vi "ActionVIOnSave.vi"(8 "error in (no error)":errorcluster, 11 "Device Item Ref in":T1 format="%.0x") -> (0 "error out":errorcluster, 3 "Device Item Ref out":T1 format="%.0x")   [LabVIEW 2019, in "Control Addon System Explorer.lvlib"]
uses:
  Control Addon System Explorer.lvlib
  <vilib>/NI VeriStand/Custom Device API/Custom Device Item Ref.ctl
  Types/Action.ctl
  Addon Shared/SubVIs/Constants.vi
  <vilib>/NI VeriStand/Custom Device API/NI VeriStand - Get Item Property.vi
  <vilib>/NI VeriStand/Custom Device API/Get Item Property (Double).vi
  <vilib>/NI VeriStand/Custom Device API/Get Item Property (Boolean).vi
  <vilib>/NI VeriStand/Custom Device API/NI VeriStand - Set Item Property.vi
  <vilib>/NI VeriStand/Custom Device API/Set Item Property (Double).vi
  <vilib>/NI VeriStand/Custom Device API/Set Item Property (Boolean).vi
  <vilib>/NI VeriStand/Custom Device Tools/Custom Device Utility Library/NI VeriStand - Search for All Items by GUID.vi
  <vilib>/NI VeriStand/Custom Device API/Get Item Property (String).vi
  <vilib>/NI VeriStand/Custom Device API/Set Item Property (String).vi
  <vilib>/NI VeriStand/Custom Device Tools/Custom Device Utility Library/Custom Device Utility Library.lvlib
  Addon Shared/Control Addon Shared.lvlib
  <vilib>/NI VeriStand/Custom Device API/Custom Device API.lvlib
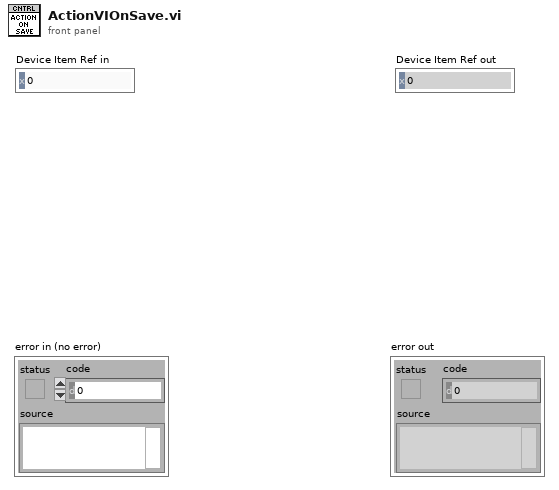
[diagram p1: front panel]
types:
  T1 = typedef "Custom Device API.lvlib/Custom Device Item Ref.ctl" = u64
  T2 = typedef "Control Addon System Explorer.lvlib/Action.ctl" = enum16{"Get", "Set"}
  T3 = typedef "Control Addon Shared.lvlib/Controller Settings.ctl" = cluster{"Output Max":dbl, "Output Min":dbl, "Setpoint Max":dbl, "Setpoint Min":dbl, "Use External Setpoint":bool, "Output Rate Limiter":dbl}
  T4 = typedef "Control Addon Shared.lvlib/PID Parameters.ctl" = cluster{"Enable Live Updates":bool, "Enable Gain Scheduling":bool, "PID Parameters":dbl[][]}
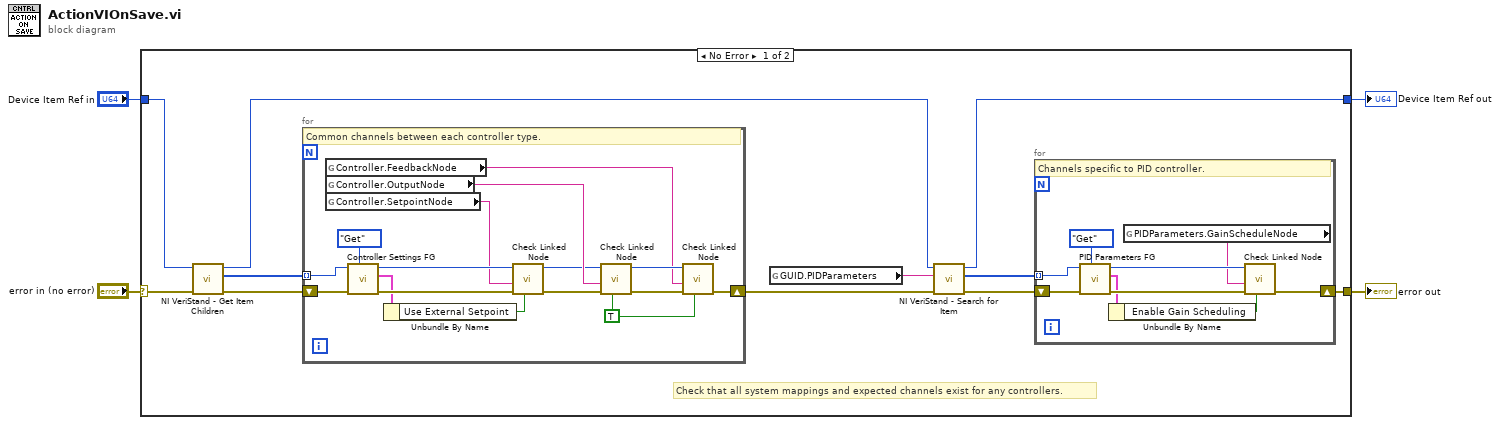
[diagram p0: block diagram]
diagram:
  n1 = case shown="No Error" "error in (no error)" {
    selector: "error in (no error)" -> [w15 w42]
    tunnel: [w5 w42] -> w3
    tunnel: "Device Item Ref in" -> [w14 w41]
    tunnel: [w6 w41] -> w1
    frame No Error {
      # "Check that all system mappings and expected channels exist for any controllers."
      n2 = call <vilib>:"NI VeriStand - Get Item Children.vi"("error in (no error)"=w15, "Item Ref in"=w14) -> ("error out"=w12:errorcluster, "Child Refs"=w13:T1[], "Item Ref out"=w7:T1)  [unwired: 6 in, 1 out]
      n3 = for {
        tunnel: w13 -> [w40] mode=indexing
        shift-right: [w25] -> w11
        shift-left: w12 -> [w36]
        w28 = TRUE ("Use Channel?")
        # "Common channels between each controller type."
        n4 = global read "Constants.vi" "Controller.FeedbackNode"() -> (w26:string)
        n5 = global read "Constants.vi" "Controller.OutputNode"() -> (w30:string)
        n6 = global read "Constants.vi" "Controller.SetpointNode"() -> (w31:string)
        n7 = call "Controller Settings FG.vi"("Action"=Action."Get", "error in (no error)"=w36, "Node Ptr"=w40) -> ("error out"=w35:errorcluster, "Controller Settings"=w33:T3, "Item Ref out"=w37:T1)  [unwired: 6 in]
        n8 = Unbundle By Name(w33) -> ("Use External Setpoint"=w32:bool)
        n9 = call "Check Linked Node.vi"("Use Channel?"=w32, "error in (no error)"=w35, "NodeName"=w31, "Item Ref in"=w37) -> ("error out"=w39:errorcluster, "Item Ref out"=w29:T1)  [unwired: 6 in]
        n10 = call "Check Linked Node.vi"("Use Channel?"=w28, "error in (no error)"=w39, "NodeName"=w30, "Item Ref in"=w29) -> ("error out"=w38:errorcluster, "Item Ref out"=w27:T1)  [unwired: 6 in]
        n11 = call "Check Linked Node.vi"("Use Channel?"=w28, "error in (no error)"=w38, "NodeName"=w26, "Item Ref in"=w27) -> ("error out"=w25:errorcluster)  [unwired: 6 in, 1 out]
      }
      n12 = global read "Constants.vi" "GUID.PIDParameters"() -> (w10:string)
      n13 = call-poly <vilib>:"NI VeriStand - Search for Item.vi"("error in"=w11, "Item GUID"=w10, "Section Ref in"=w7) -> ("error out"=w9:errorcluster, "Item Refs"=w8:T1[], "Section Ref out"=w6:T1)  [unwired: 5 in, 1 out]
      n14 = for {
        tunnel: w8 -> [w24] mode=indexing
        shift-right: [w16] -> w5
        shift-left: w9 -> [w22]
        # "Channels specific to PID controller."
        n15 = call "PID Parameters FG.vi"("Action"=Action."Get", "error in (no error)"=w22, "Node Ptr"=w24) -> ("error out"=w21:errorcluster, "Parameters"=w19:T4, "Item Ref out"=w23:T1)  [unwired: 6 in]
        n16 = Unbundle By Name(w19) -> ("Enable Gain Scheduling"=w18:bool)
        n17 = global read "Constants.vi" "PIDParameters.GainScheduleNode"() -> (w17:string)
        n18 = call "Check Linked Node.vi"("Use Channel?"=w18, "error in (no error)"=w21, "NodeName"=w17, "Item Ref in"=w23) -> ("error out"=w16:errorcluster)  [unwired: 6 in, 1 out]
      }
    }
    frame Error {
    }
  }
  "error out" <- w3
  "Device Item Ref out" <- w1
